vi "List Log Data.vi"(8 "error in (no error)":errorcluster, 10 "Data Queue":refnum<queue>, 11 "Logging Configuration":T1) -> (0 "error out":errorcluster)   [LabVIEW 2022 SP3, in "Logging.lvlib"]
doc: "This VI uses the TDMS Write function to write data to a TDMS file."
uses:
  Logging.lvlib
  Logging Configuration.ctl
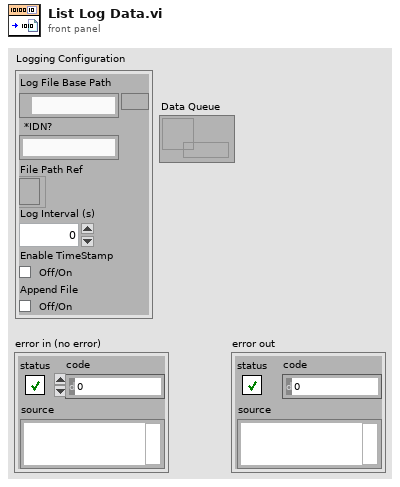
[diagram p1: front panel]
types:
  T1 = typedef "Logging.lvlib/Logging Configuration.ctl" = cluster{"Log File Base Path":path, "*IDN?":string, "File Path Ref":refnum<file>, "Log Interval (s)":dbl, "Enable TimeStamp":bool, "Append File":bool}
  T2 = enum16{"open", "replace", "create", "open or create", "replace or create", "replace or create with confirmation"}
  T3 = cluster{"Numeric":dbl, "Numeric":dbl, "Numeric":dbl, timestamp}
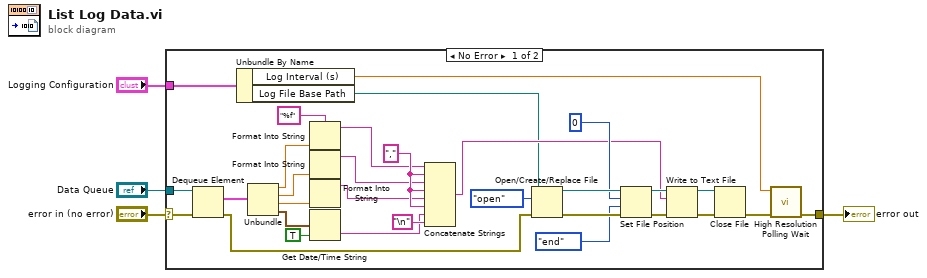
[diagram p0: block diagram]
diagram:
  n1 = case shown="No Error" "error in (no error)" {
    selector: "error in (no error)" -> [w34 w36]
    tunnel: "Logging Configuration" -> [w35 _]
    tunnel: [w7 w36] -> w3
    tunnel: "Data Queue" -> [w5 _]
    frame No Error {
      w19 = ","
      w15 = "%f"
      n2 = Dequeue Element(queue=w5, error in (no error)=w34) -> (element=w33:T3, error out=w12:errorcluster)  [unwired: 1 in, 2 out]
      n3 = Unbundle By Name(w35) -> ("Log Interval (s)"=w6:dbl, "Log File Base Path"=w13:path)
      n4 = Unbundle(w33) -> ("Numeric"=w20:dbl, "Numeric"=w21:dbl, "Numeric"=w22:dbl, w11:timestamp)
      n5 = Format Into String(format string=w15, w20) -> (resulting string=w18:string)  [unwired: 2 in, 1 out]
      n6 = Format Into String(format string=w15, w21) -> (resulting string=w17:string)  [unwired: 2 in, 1 out]
      n7 = Format Into String(format string=w15, w22) -> (resulting string=w16:string)  [unwired: 2 in, 1 out]
      n8 = Get Date/Time String(seconds (now)=w11, want seconds? (F)=TRUE) -> (time string=w9:string)  [unwired: 1 in, 1 out]
      n9 = Concatenate Strings(w18, w19, w17, w19, w16, w19, w9, "\n") -> (w23:string)
      n10 = Open/Create/Replace File(file path (use dialog)=w13, error in=w12, operation (0:open)=T2."open") -> (refnum out=w29:refnum<file>, error out=w27:errorcluster)  [unwired: 3 in, 1 out]
      n11 = Set File Position(offset (in bytes) (0)=i64 0, refnum=w29, from (0:start)=enum16{"start", "end", "current"}."end", error in=w27) -> (refnum out=w28:refnum<file>, error out=w26:errorcluster)
      n12 = Write to Text File(file (use dialog)=w28, text=w23, error in=w26) -> (refnum out=w31:refnum<file>, error out=w32:errorcluster)  [unwired: 1 in, 1 out]
      n13 = Close File(refnum=w31, error in=w32) -> (error out=w8:errorcluster)  [unwired: 1 out]
      n14 = call <vilib>:"High Resolution Polling Wait.vi"("error in (no error)"=w8, "seconds to wait"=w6) -> ("error out"=w7:errorcluster)  [unwired: 9 in]
    }
    frame Error {
    }
  }
  "error out" <- w3
